vi "Module ID.vi"(11 "GUI Helper in":refnum<class "GUI Helper.lvclass">) -> (2 "Module ID":string)   [LabVIEW 2020, in "VolatusGUI.lvlib" / "GUI Helper.lvclass"]
uses:
  GUI Helper.lvclass
  GUI Helper.lvclass/GUI Helper.ctl
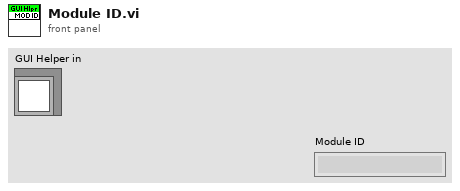
[diagram p1: front panel]
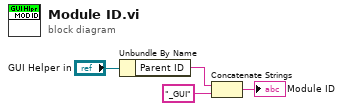
[diagram p0: block diagram]
diagram:
  n1 = Unbundle By Name("GUI Helper in") -> ("Parent ID"=w3:string)
  n2 = Concatenate Strings(w3, "_GUI" ("string")) -> (→"Module ID":string)
